vi "While loop.vi"() -> ()   [LabVIEW 2011]
panel:
  out "Array":dbl[](array[numeric])
  out "Factorial":dbl
  in  "Number":dbl
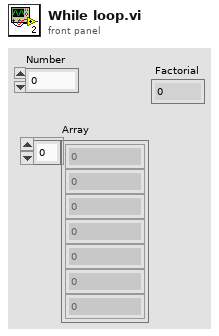
[diagram p1: front panel]
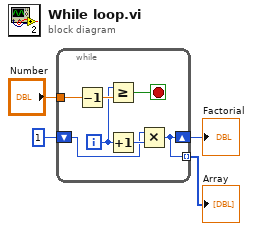
[diagram p0: block diagram]
diagram:
  n1 = while {
    tunnel: "Number" -> [w11]
    shift-right: [w5] -> w1
    shift-left: 1 -> [w6]
    tunnel: [w5] -> w2 mode=indexing
    i -> [w8]
    stop <- w10 stop-if-true
    n2 = Decrement(x=w11) -> (x-1=w9:dbl)
    n3 = Greater Or Equal?(x=w8, y=w9) -> (x >= y?=w10:bool)
    n4 = Increment(x=w8) -> (x+1=w7:i32)
    n5 = Multiply(x=w6, y=w7) -> (x*y=w5:i32)
  }
  "Factorial" <- w1
  "Array" <- w2
